vi "FPGA_AnalogTriggerWriteConfiguration.vi"(8 "error in (no error)":errorcluster, 10 "AnalogTriggerSource":T1={"Channel"=enum."AI 1", "Averaged"=FALSE, "Filter"=FALSE}, 11 "AnalogTriggerDevRef":T3) -> (0 "error out":errorcluster, 3 "AnalogTriggerDevRef":T3)   [LabVIEW 2017]
uses:
  <vilib>/Rock Robotics/SystemInterfaces/AnalogTrigger/FPGA_AnalogTriggerDevRef.ctl
  <vilib>/Rock Robotics/SystemInterfaces/AnalogTrigger/FPGA_AnalogTriggerIndex.ctl
  <vilib>/Rock Robotics/SystemInterfaces/AnalogTrigger/FPGA_AnalogTriggerSource.ctl
  <vilib>/Rock Robotics/SystemInterfaces/AI/FPGA_AIChannel.ctl
  <vilib>/rvi/errors/niLvFpgaAdjustHostInterfaceError.vi
  <vilib>/Utility/error.llb/Error Cluster From Error Code.vi
  <vilib>/Rock Robotics/SystemInterfaces/System/FPGA_SystemFPGA Ref Global.vi
  <vilib>/Rock Robotics/SystemInterfaces/System/FPGA_SystemFRC FPGA Ref.ctl
  <vilib>/rvi/interface/nirviReadWriteControl/nirviReadWriteControl.xnode
  NiFpgaLv.dll
  <vilib>/rvi/interface/Simulation/niFpgaSimulationCallBeginRW.vi
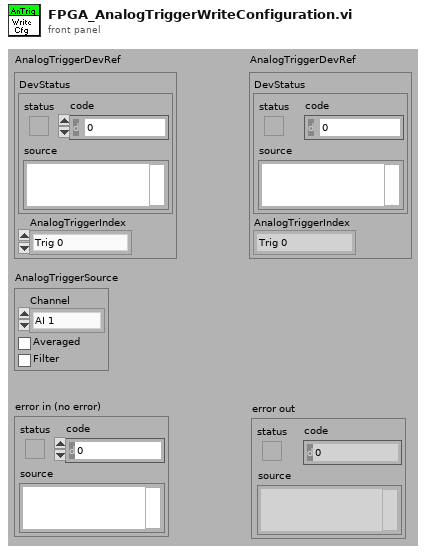
[diagram p1: front panel]
types:
  T1 = typedef "FPGA_AnalogTriggerSource.ctl" = cluster{"Channel":T2, "Averaged":bool, "Filter":bool}
  T2 = typedef "FPGA_AIChannel.ctl" = enum8{"AI 0", "AI 1", "AI 2", "AI 3", "AI MXP 0", "AI MXP 1", "AI MXP 2", "AI MXP 3", "Invalid"}
  T3 = typedef "FPGA_AnalogTriggerDevRef.ctl" = cluster{"DevStatus":errorcluster, "AnalogTriggerIndex":T4}
  T4 = typedef "FPGA_AnalogTriggerIndex.ctl" = enum8{"Trig 0", "Trig 1", "Trig 2", "Trig 3", "Trig 4", "Trig 5", "Trig 6", "Trig 7", "Invalid"}
  T5 = typedef "FPGA_SystemFRC FPGA Ref.ctl" = refnum<k20>
  T6 = cluster{"Channel":fxp<+,3,3>, "Averaged":bool, "Filter":bool, "FloatingRollover":bool, "RolloverLimit":fxp<+/-,8,12>}
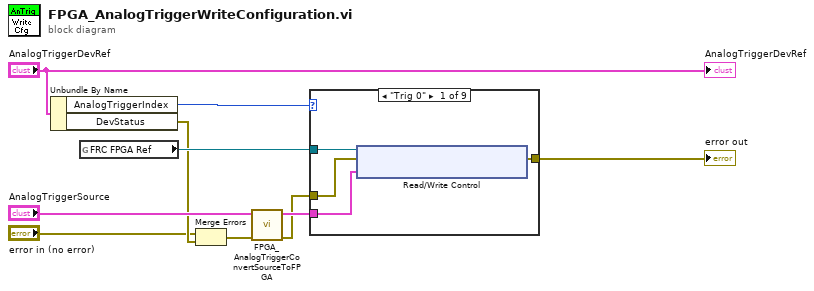
[diagram p0: block diagram]
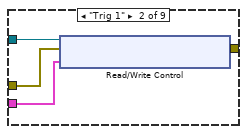
[diagram p2: hidden frame]
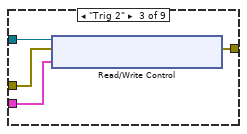
[diagram p3: hidden frame]
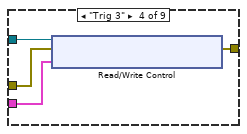
[diagram p4: hidden frame]
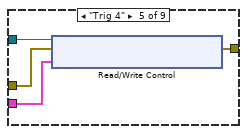
[diagram p5: hidden frame]
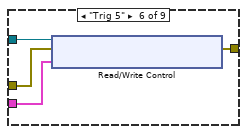
[diagram p6: hidden frame]
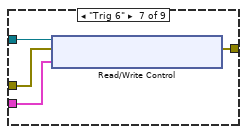
[diagram p7: hidden frame]
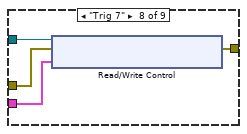
[diagram p8: hidden frame]
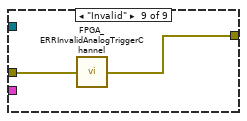
[diagram p9: hidden frame]
diagram:
  n1 = Unbundle By Name("AnalogTriggerDevRef") -> ("AnalogTriggerIndex"=w7:T4, "DevStatus"=w3:errorcluster)
  n2 = global read "FPGA_SystemFPGA Ref Global.vi" "FRC FPGA Ref"() -> (w4:T5)
  n3 = Merge Errors("error in (no error)", w3) -> (w1:errorcluster)
  n4 = call <vilib>:"FPGA_AnalogTriggerConvertSourceToFPGA.vi"("error in (no error)"=w1, "AnalogTriggerSource"="AnalogTriggerSource") -> ("error out"=w5:errorcluster, "FPGASourceType"=w6:T6)  [unwired: 8 out]
  n5 = case shown="\"Trig 0\"" w7 {
    tunnel: w4 -> [w14 w18 w22 w26 w30 w34 w38 w42 _]
    tunnel: [w13 w17 w21 w25 w29 w33 w37 w41 w43] -> w10
    tunnel: w6 -> [w11 w15 w19 w24 w28 w32 w36 w40 _]
    tunnel: w5 -> [w12 w16 w20 w23 w27 w31 w35 w39 w44]
    frame "Trig 0" {
      n6 = xnode "Read/Write Control"("FPGA VI Reference In"=w14, "error in"=w12, "AnalogTrigger0.SourceSelect"=w11) -> ("error out"=w13:errorcluster)  [unwired: 1 out]
    }
    frame "Trig 1" {
      n7 = xnode "Read/Write Control"("FPGA VI Reference In"=w18, "error in"=w16, "AnalogTrigger1.SourceSelect"=w15) -> ("error out"=w17:errorcluster)  [unwired: 1 out]
    }
    frame "Trig 2" {
      n8 = xnode "Read/Write Control"("FPGA VI Reference In"=w22, "error in"=w20, "AnalogTrigger2.SourceSelect"=w19) -> ("error out"=w21:errorcluster)  [unwired: 1 out]
    }
    frame "Trig 3" {
      n9 = xnode "Read/Write Control"("FPGA VI Reference In"=w26, "error in"=w23, "AnalogTrigger3.SourceSelect"=w24) -> ("error out"=w25:errorcluster)  [unwired: 1 out]
    }
    frame "Trig 4" {
      n10 = xnode "Read/Write Control"("FPGA VI Reference In"=w30, "error in"=w27, "AnalogTrigger4.SourceSelect"=w28) -> ("error out"=w29:errorcluster)  [unwired: 1 out]
    }
    frame "Trig 5" {
      n11 = xnode "Read/Write Control"("FPGA VI Reference In"=w34, "error in"=w31, "AnalogTrigger5.SourceSelect"=w32) -> ("error out"=w33:errorcluster)  [unwired: 1 out]
    }
    frame "Trig 6" {
      n12 = xnode "Read/Write Control"("FPGA VI Reference In"=w38, "error in"=w35, "AnalogTrigger6.SourceSelect"=w36) -> ("error out"=w37:errorcluster)  [unwired: 1 out]
    }
    frame "Trig 7" {
      n13 = xnode "Read/Write Control"("FPGA VI Reference In"=w42, "error in"=w39, "AnalogTrigger7.SourceSelect"=w40) -> ("error out"=w41:errorcluster)  [unwired: 1 out]
    }
    frame "Invalid" {
      n14 = call <vilib>:"FPGA_ERRInvalidAnalogTriggerChannel.vi"("error in (no error)"=w44) -> ("error out"=w43:errorcluster)
    }
  }
  "error out" <- w10
  "AnalogTriggerDevRef" <- "AnalogTriggerDevRef"
